vi "create_NG_folder.vi"(11 "output folder in":path) -> (3 "NG folder array":string[](array[string]))   [LabVIEW 2017]
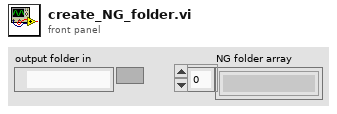
[diagram p1: front panel]
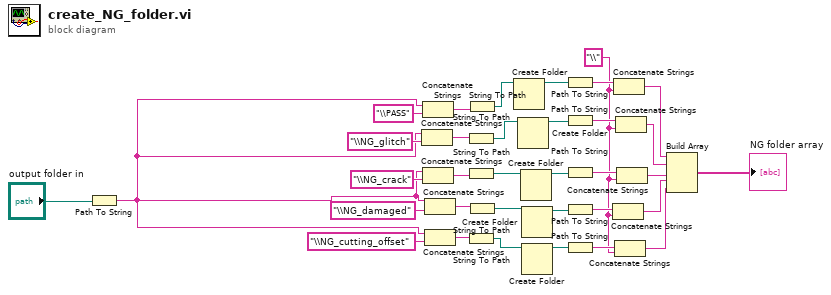
[diagram p0: block diagram]
diagram:
  w5 = "\\" ("string")
  n1 = Path To String(path="output folder in") -> (string=w17:string)
  n2 = Concatenate Strings(w17, "\\NG_glitch" ("string")) -> (w26:string)
  n3 = Concatenate Strings(w17, "\\PASS" ("string")) -> (w20:string)
  n4 = Concatenate Strings(w17, "\\NG_crack" ("string")) -> (w28:string)
  n5 = Concatenate Strings(w17, "\\NG_damaged" ("string")) -> (w29:string)
  n6 = Concatenate Strings(w17, "\\NG_cutting_offset" ("string")) -> (w30:string)
  n7 = String To Path(string=w26) -> (path=w27:path)
  n8 = String To Path(string=w28) -> (path=w31:path)
  n9 = String To Path(string=w30) -> (path=w33:path)
  n10 = String To Path(string=w20) -> (path=w19:path)
  n11 = String To Path(string=w29) -> (path=w32:path)
  n12 = Create Folder(path (use dialog)=w19) -> (created path=w16:path)  [unwired: 2 in, 2 out]
  n13 = Create Folder(path (use dialog)=w27) -> (created path=w15:path)  [unwired: 2 in, 2 out]
  n14 = Create Folder(path (use dialog)=w31) -> (created path=w14:path)  [unwired: 2 in, 2 out]
  n15 = Create Folder(path (use dialog)=w32) -> (created path=w13:path)  [unwired: 2 in, 2 out]
  n16 = Create Folder(path (use dialog)=w33) -> (created path=w12:path)  [unwired: 2 in, 2 out]
  n17 = Path To String(path=w16) -> (string=w11:string)
  n18 = Path To String(path=w15) -> (string=w9:string)
  n19 = Path To String(path=w14) -> (string=w8:string)
  n20 = Path To String(path=w13) -> (string=w7:string)
  n21 = Path To String(path=w12) -> (string=w6:string)
  n22 = Concatenate Strings(w7, w5) -> (w2:string)
  n23 = Concatenate Strings(w11, w5) -> (w4:string)
  n24 = Concatenate Strings(w6, w5) -> (w1:string)
  n25 = Concatenate Strings(w9, w5) -> (w3:string)
  n26 = Concatenate Strings(w8, w5) -> (w10:string)
  n27 = Build Array(w4, w3, w10, w2, w1) -> (→"NG folder array":string[])
